vi "ReadFreeRunningCounter.vi"(7 "Address Space":T1=12 items=["VXI/VME A16"=1, "VXI/VME A24"=2, "VXI/VME A32"=3, "VXI/VME A64"=4, "PXI Memory Allocations"=9, "PXI Configuration"=10, "PXI BAR0"=11, "PXI BAR1"=12, "PXI BAR2"=13, "PXI BAR3"=14, "PXI BAR4"=15, "PXI BAR5"=16], 8 "error in":errorcluster, 9 "Save Register Address":u32=2076 format="%x", 11 "VISA resource name":refnum<visa-resource-name>) -> (0 "error out":errorcluster, 3 "Counter Data":u32)   [LabVIEW 2014]
uses:
  <vilib>/Instr/_visa.llb/VISA Register Access Address Space.ctl
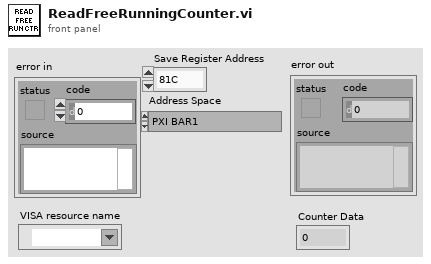
[diagram p1: front panel]
types:
  T1 = typedef "VISA Register Access Address Space.ctl" = u16
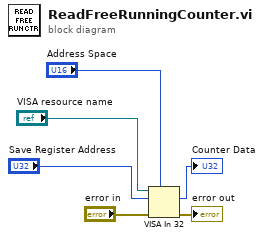
[diagram p0: block diagram]
diagram:
  n1 = VISA In 32(7:"Address Space", 8:"error in", 10:"Save Register Address", 11:"VISA resource name") -> (0:→"error out":errorcluster, 2:→"Counter Data":u32)  [unwired: 1 out]
